vi "AO-handler.vi"(9 "Analog Outputs Ctrl":T1, 11 "Analog Output State":T1) -> (0 "output state changed":bool, 2 "hex integer string":string, 3 "Analog Outputs":T1, 4 "number":u32, 6 "Analog Val array":dbl[](array[numeric]))   [LabVIEW 2020]
uses:
  controls/analog-output-cluster.ctl
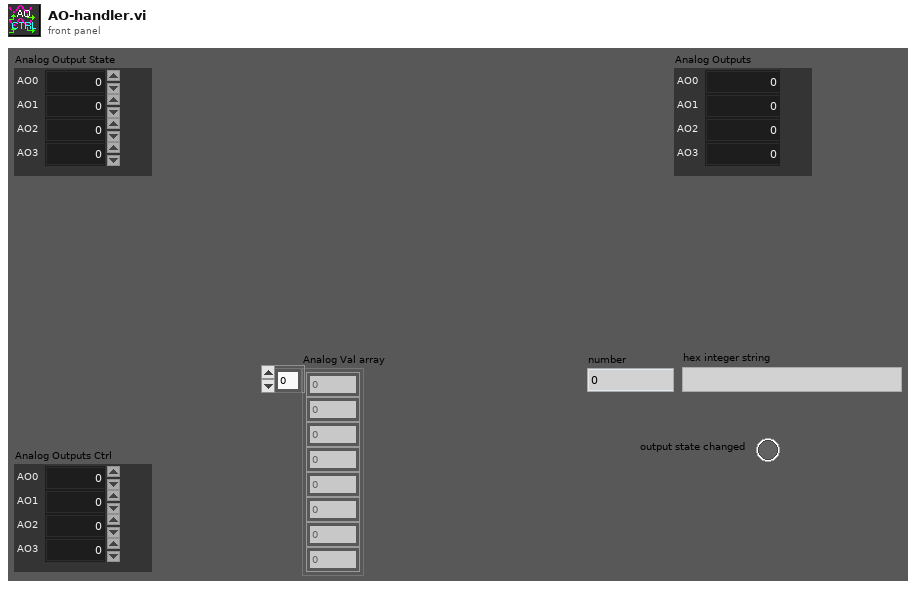
[diagram p1: front panel]
types:
  T1 = typedef "analog-output-cluster.ctl" = cluster{"AO0":dbl, "AO1":dbl, "AO2":dbl, "AO3":dbl}
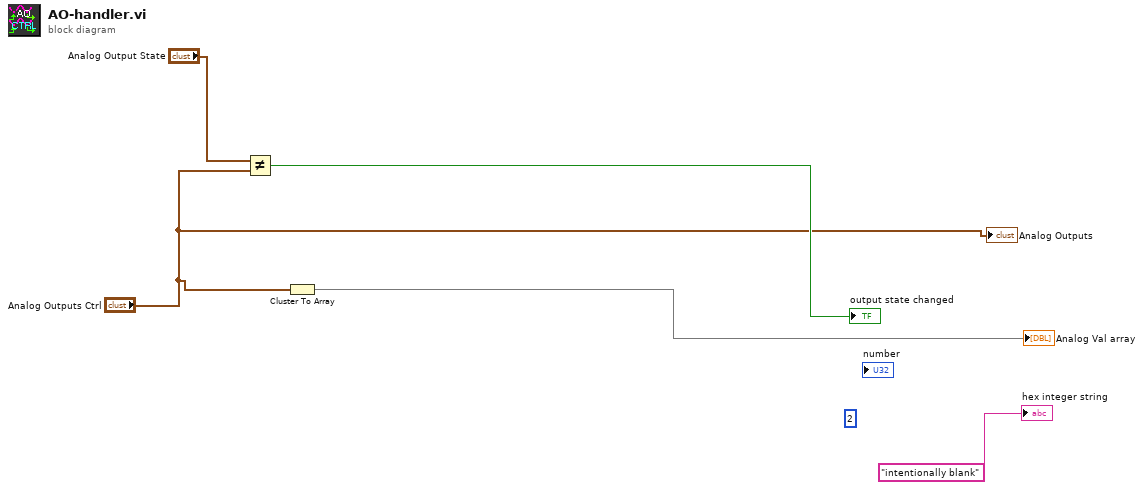
[diagram p0: block diagram]
diagram:
  (unwired) i16 2 ("width (-)")
  n1 = Not Equal?(x="Analog Output State", y="Analog Outputs Ctrl") -> (x != y?=→"output state changed":bool)
  n2 = Cluster To Array(cluster="Analog Outputs Ctrl") -> (array=→"Analog Val array":dbl[])
  "hex integer string" <- "intentionally blank" ("hex integer string")
  "Analog Outputs" <- "Analog Outputs Ctrl"
